vi "FTW-Example-Actors.vi"() -> ()   [LabVIEW 2013]
uses:
  src/core/actor/connector/FTW-Actor-Connector.lvclass
panel:
  out "Actor Pool Spawn":dbl format="Actor Pool Spawn: %_3psec"
  out "Overall Pass?":bool
  out "Total Elapsed Time":dbl format="Total Test Time: %_3psec"
  out "\"FTW: Ping\" Times":cluster{dbl[]}[](graph)
  out "Results":T1(array[cluster])
  in  "Test to Perform":T2(radio)=enum."Parallel: 10x10"
  out "\"PING\" Times":cluster{dbl[]}[](graph)
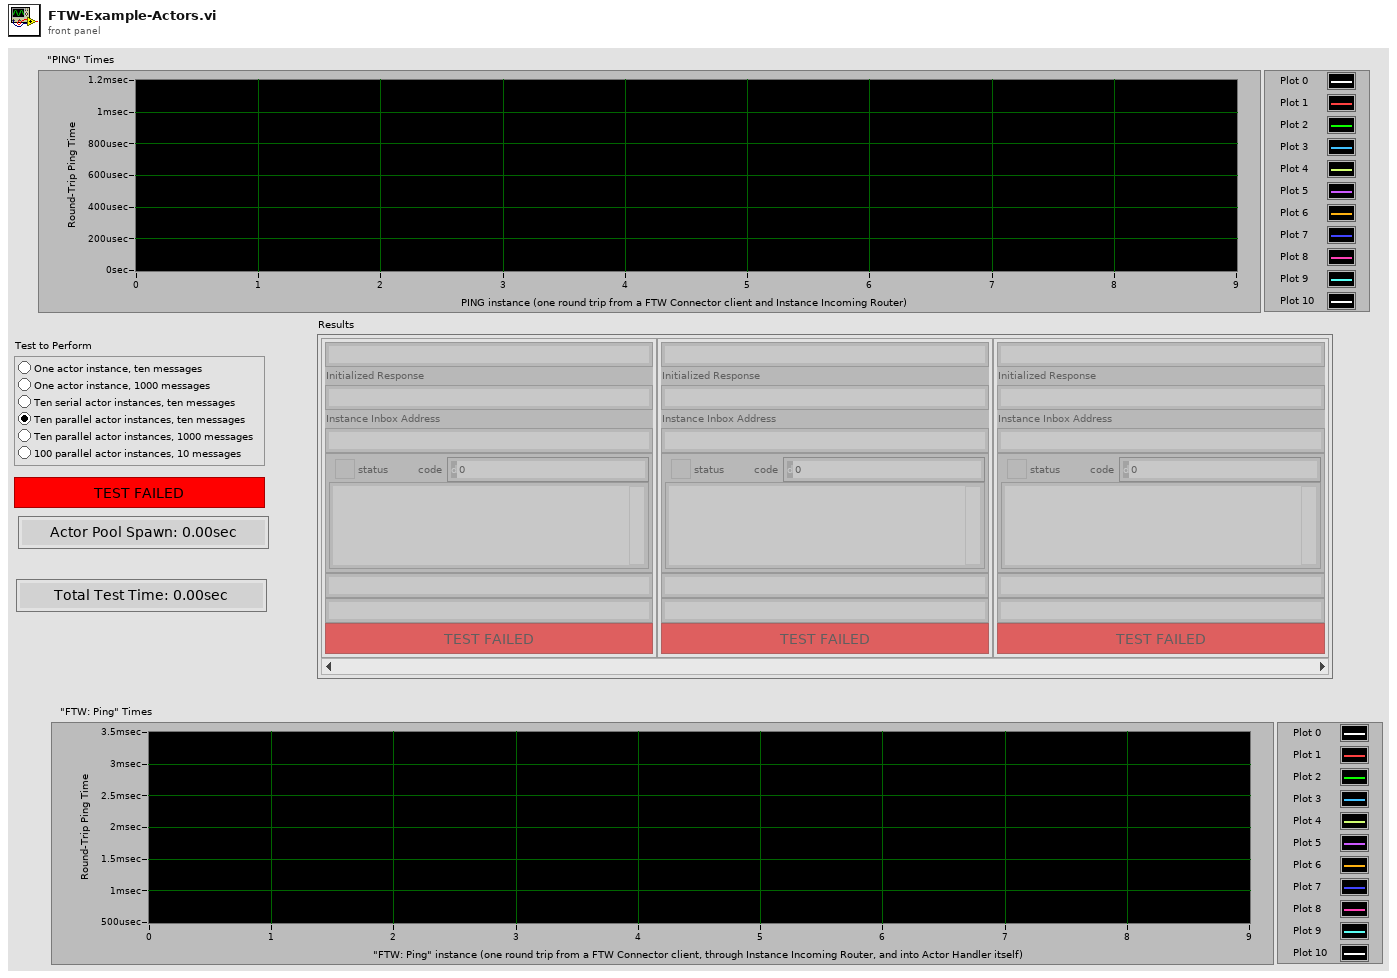
[diagram p1: front panel]
types:
  T1 = cluster{"Server Address":string, "Initialized Response":string, "Instance Inbox Address":string, "Error":errorcluster, "Server Address":string, "Server Address":string, "Pass?":bool}[]
  T2 = enum32{"Serial: 1x10", "Serial: 1x1000", "Serial: 10x10", "Parallel: 10x10", "Parallel: 10x100", "Parallel: 100x10"}
  T3 = cluster{i32, "Initialized Response":string, "Instance Inbox Address":string, "Instance Publisher Address":string, "error out":errorcluster}
  T4 = cluster{i32, bool, bool, "Timed out?":bool, cluster{dbl[]}, cluster{dbl[]}, "error out":errorcluster}
  T5 = cluster{string, "Initialized Response":string, "Instance Inbox Address":string, "error out":errorcluster, string, string, bool}
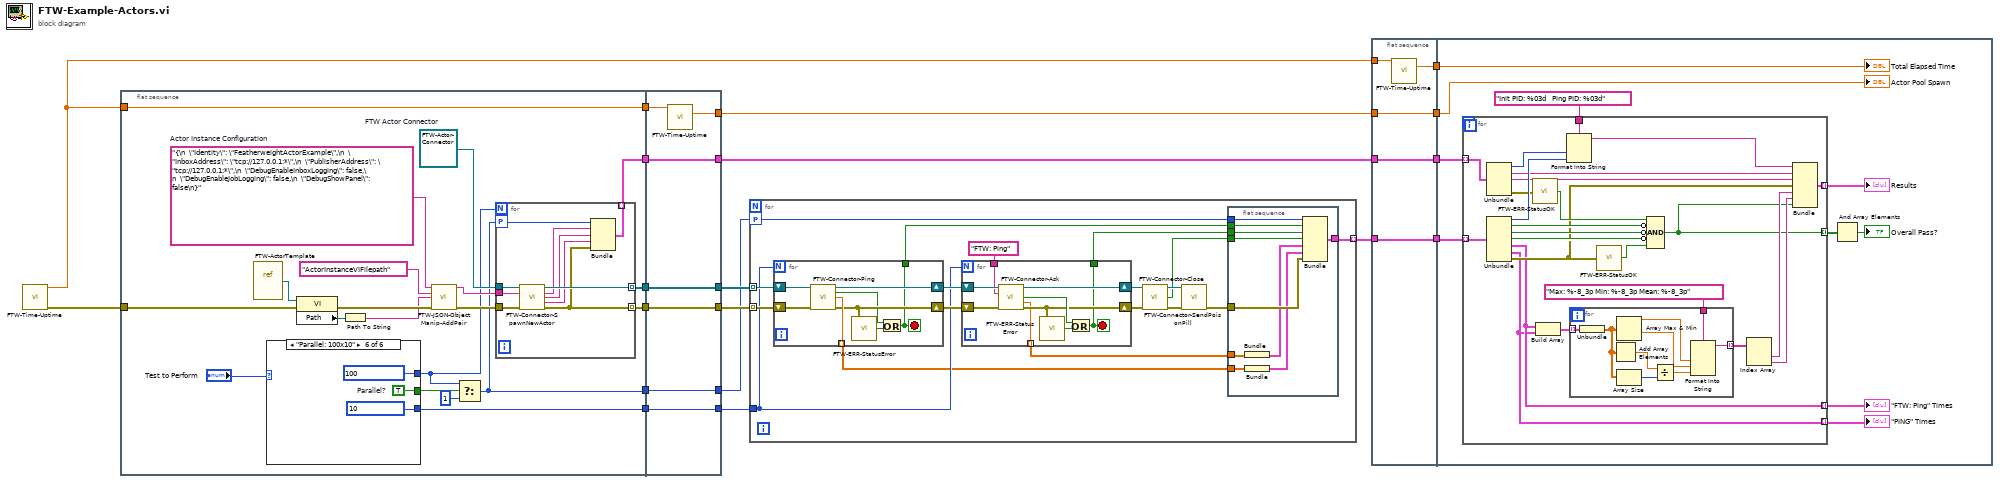
[diagram p0: block diagram]
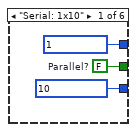
[diagram p2: hidden frame]
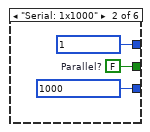
[diagram p3: hidden frame]
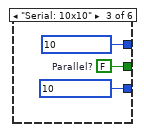
[diagram p4: hidden frame]
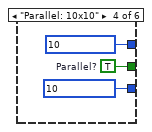
[diagram p5: hidden frame]
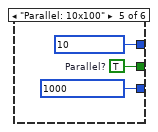
[diagram p6: hidden frame]
diagram:
  n1 = call "FTW-Time-Uptime.vi"() -> ("Current Uptime"=w4:dbl, "error out"=w13:errorcluster)  [unwired: 13 in, 1 out]
  n2 = flat-sequence {
    tunnel: w13 -> [w21]
    tunnel: [w30] -> w9
    tunnel: [w29] -> w8
    tunnel: [w27] -> w7
    tunnel: [w23] -> w6
    tunnel: [w22] -> w5
    tunnel: w4 -> [w20]
    tunnel: [w20] -> w3
    tunnel: [w70] -> w15
    tunnel: [w71] -> w16
    tunnel: [w72] -> w17
    tunnel: [w73] -> w18
    tunnel: [w74] -> w19
    tunnel: w9 -> [w74]
    tunnel: w8 -> [w73]
    tunnel: w7 -> [w72]
    tunnel: w6 -> [w71]
    tunnel: w5 -> [w70]
    tunnel: w3 -> [w69]
    tunnel: [w68] -> w1
    frame #0 {
      w37 = "{\n  \"Identity\": \"FeatherweightActorExample\",\n  \"InboxAddress\": \"tcp://127.0.0.1:*\",\n  \"PublisherAddress\": \"tcp://127.0.0.1:*\",\n  \"DebugEnableInboxLogging\": false,\n  \"DebugEnableJobLogging\": false,\n  \"DebugShowPanel\": false\n}"  # Actor Instance Configuration
      w39 = refnum<class "FTW-Actor-Connector.lvclass"> refnum  # FTW Actor Connector
      n3 = vi-ref "FTW-ActorTemplate.vi"() -> (w38:refnum<vi>)
      n4 = case shown="\"Parallel: 100x10\"" "Test to Perform" {
        tunnel: [1 1 10 10 10 100] -> w26
        tunnel: [10 1000 10 10 1000 10] -> w27
        tunnel: [w50 w53 w56 w59 w62 w65] -> w25
        frame "Serial: 1x10" {
          w50 = FALSE  # Parallel?
        }
        frame "Serial: 1x1000" {
          w53 = FALSE  # Parallel?
        }
        frame "Serial: 10x10" {
          w56 = FALSE  # Parallel?
        }
        frame "Parallel: 10x10" {
          w59 = TRUE  # Parallel?
        }
        frame "Parallel: 10x100" {
          w62 = TRUE  # Parallel?
        }
        frame "Parallel: 100x10" {
          w65 = TRUE  # Parallel?
        }
      }
      n5 = property class="VI"(reference=w38, error in=w21) -> (error out=w35:errorcluster, "Path"=w32:path)  [unwired: 1 out]
      n6 = Path To String(path=w32) -> (string=w31:string)
      n7 = call "FTW-JSON-ObjectManip-AddPair.vi"("Input JSON Object"=w37, "Key"="ActorInstanceVIFilepath", "Value"=w31, "error in"=w35) -> ("Output JSON Object"=w36:string, "error out"=w34:errorcluster)  [unwired: 10 in]
      n8 = Select(t=w26, s=w25, f=1) -> (s? t:f=w23:i32)
      n9 = for {
        N: w26 -> [_]
        tunnel: w39 -> [w49]
        tunnel: w36 -> [w48]
        tunnel: w34 -> [w47]
        tunnel: [w46] -> w30 mode=indexing
        tunnel: [w41] -> w29 mode=indexing
        tunnel: [w42] -> w22 mode=indexing
        workers-P: w23 -> [w40]
        n10 = call "FTW-Connector-SpawnNewActor.vi"("FTW Actor Connector Type"=w49, "Instance Configuration"=w48, "error in"=w47) -> ("FTW Actor Connector"=w46:refnum<class "FTW-Actor-Connector.lvclass">, "Initialized Response"=w45:string, "Instance Inbox Address"=w44:string, "Instance Publisher Address"=w43:string, "error out"=w41:errorcluster)  [unwired: 8 in]
        n11 = Bundle(w40, "Initialized Response"=w45, "Instance Inbox Address"=w44, "Instance Publisher Address"=w43, "error out"=w41) -> (w42:T3)  [unwired: 1 in]
      }
    }
    frame #1 {
      n12 = call "FTW-Time-Uptime.vi"("Previous Uptime"=w69) -> ("Elapsed Time"=w68:dbl)  [unwired: 12 in, 2 out]
    }
  }
  n13 = for {
    tunnel: w19 -> [w90] mode=indexing
    tunnel: w18 -> [w89] mode=indexing
    tunnel: w17 -> [w83]
    workers-P: w16 -> [w82]
    tunnel: [w79] -> w14 mode=indexing
    n14 = for {
      N: w83 -> [_]
      tunnel: [w116] -> w75 mode=indexing
      shift-right: [w117] -> w87
      shift-left: w90 -> [w119]
      shift-right: [w115] -> w86
      shift-left: w89 -> [w118]
      tunnel: [w112] -> w81
      stop <- w112 stop-if-true
      n15 = call-dynamic "FTW-Connector-Ping.vi"("FTW Actor Connector Type"=w119, "error in"=w118) -> ("FTW Actor Connector"=w117:refnum<class "FTW-Actor-Connector.lvclass">, "Timed out?"=w113:bool, "Roundtrip Time"=w116:dbl, "error out"=w115:errorcluster)  [unwired: 10 in]
      n16 = call "FTW-ERR-StatusError.vi"("error to check"=w115) -> ("Error?"=w114:bool)
      n17 = Or(x=w113, y=w114) -> (x .or. y?=w112:bool)
    }
    n18 = for {
      N: w83 -> [_]
      tunnel: [w106] -> w76 mode=indexing
      shift-right: [w109] -> w85
      shift-left: w87 -> [w110]
      shift-right: [w107] -> w84
      shift-left: w86 -> [w105]
      tunnel: "FTW: Ping" ("Request Header") -> [w104]
      tunnel: [w103] -> w80
      stop <- w103 stop-if-true
      n19 = call "FTW-Connector-Ask.vi"("FTW Actor Connector"=w110, "Request Header"=w104, "error in"=w105) -> ("FTW Actor Connector out"=w109:refnum<class "FTW-Actor-Connector.lvclass">, "Timed out?"=w108:bool, "Roundtrip Time"=w106:dbl, "error out"=w107:errorcluster)  [unwired: 8 in, 1 out]
      n20 = call "FTW-ERR-StatusError.vi"("error to check"=w107) -> ("Error?"=w111:bool)
      n21 = Or(x=w108, y=w111) -> (x .or. y?=w103:bool)
    }
    n22 = call-dynamic "FTW-Connector-SendPoisonPill.vi"("FTW Actor Connector"=w85, "error in"=w84) -> ("FTW Actor Connector out"=w92:refnum<class "FTW-Actor-Connector.lvclass">, "Timed out?"=w78:bool, "error out"=w91:errorcluster)  [unwired: 10 in, 1 out]
    n23 = call-dynamic "FTW-Connector-Close.vi"("FTW Actor Connector"=w92, "error in"=w91) -> ("error out"=w77:errorcluster)  [unwired: 13 in]
    n24 = flat-sequence {
      tunnel: w82 -> [w102]
      tunnel: w81 -> [w101]
      tunnel: w80 -> [w100]
      tunnel: [w99] -> w79
      tunnel: w78 -> [w98]
      tunnel: w77 -> [w97]
      tunnel: w76 -> [w95]
      tunnel: w75 -> [w93]
      frame #0 {
        n25 = Bundle(w95) -> (w96:cluster{dbl[]})  [unwired: 1 in]
        n26 = Bundle(w93) -> (w94:cluster{dbl[]})  [unwired: 1 in]
        n27 = Bundle(w102, w101, w100, "Timed out?"=w98, w96, w94, "error out"=w97) -> (w99:T4)  [unwired: 1 in]
      }
    }
  }
  n28 = flat-sequence {
    tunnel: w14 -> [w123]
    tunnel: w15 -> [w124]
    tunnel: [w124] -> w12
    tunnel: [w123] -> w11
    tunnel: w4 -> [w122]
    tunnel: [w121] -> w10
    tunnel: [w120] -> w2
    tunnel: w1 -> [w120]
    tunnel: w12 -> [w134]
    tunnel: w11 -> [w133]
    tunnel: w10 -> [w128]
    tunnel: w2 -> [w125]
    frame #0 {
      n29 = call "FTW-Time-Uptime.vi"("Previous Uptime"=w122) -> ("Elapsed Time"=w121:dbl)  [unwired: 12 in, 2 out]
    }
    frame #1 {
      n30 = for {
        tunnel: w134 -> [w158] mode=indexing
        tunnel: w133 -> [w157] mode=indexing
        tunnel: "Init PID: %03d   Ping PID: %03d" ("format string") -> [w156]
        tunnel: [w139] -> w131 mode=indexing
        tunnel: [w138] -> w130 mode=indexing
        tunnel: [w137] -> w129 mode=indexing
        tunnel: [w136] -> w127 mode=indexing
        n31 = Unbundle(w158) -> (w155:i32, "Initialized Response"=w146:string, "Instance Inbox Address"=w145:string, "error out"=w153:errorcluster)  [unwired: 1 out]
        n32 = Unbundle(w157) -> (w154:i32, w151:bool, w150:bool, "Timed out?"=w149:bool, w138:cluster{dbl[]}, w137:cluster{dbl[]}, "error out"=w144:errorcluster)
        n33 = call "FTW-ERR-StatusOK.vi"("error to check"=w153) -> ("Status OK?"=w152:bool)
        n34 = Build Array(w138, w137) -> (w143:cluster{dbl[]}[])
        n35 = Format Into String(format string=w156, w155, w154) -> (resulting string=w147:string)  [unwired: 2 in, 1 out]
        n36 = for {
          tunnel: w143 -> [w162] mode=indexing
          tunnel: [w160] -> w142 mode=indexing
          tunnel: "Max: %-8_3p Min: %-8_3p Mean: %-8_3p" ("format string") -> [w159]
          n37 = Unbundle(w162) -> (w161:dbl[])
          n38 = Add Array Elements(numeric array=w161) -> (sum=w167:dbl)
          n39 = Array Max & Min(array=w161) -> (max value=w165:dbl, min value=w164:dbl)  [unwired: 2 out]
          n40 = Array Size(array=w161) -> (size(s)=w166:i32)
          n41 = Divide(x=w167, y=w166) -> (x/y=w163:dbl)
          n42 = Format Into String(format string=w159, w165, w164, w163) -> (resulting string=w160:string)  [unwired: 2 in, 1 out]
        }
        n43 = call "FTW-ERR-StatusOK.vi"("error to check"=w144) -> ("Status OK?"=w148:bool)
        n44 = Compound Arithmetic op=AND(w152, invert w151, invert w150, invert w149, w148) -> (w136:bool)
        n45 = Index Array(array=w142) -> (element #1=w141:string, element #2=w140:string)  [unwired: 2 in]
        n46 = Bundle(w147, "Initialized Response"=w146, "Instance Inbox Address"=w145, "error out"=w144, w141, w140, w136) -> (w139:T5)  [unwired: 1 in]
      }
      "\"PING\" Times" <- w129
      "Results" <- w131
      "\"FTW: Ping\" Times" <- w130
      n47 = And Array Elements(Boolean array=w127) -> (logical AND=→"Overall Pass?":bool)
      "Total Elapsed Time" <- w128
      "Actor Pool Spawn" <- w125
    }
  }
